vi "Read_Flatten.vi"(8 "error in":errorcluster, 11 "ChillerNew.lvclass":refnum<class "ChillerNew.lvclass">) -> (0 "error out":errorcluster, 2 "ReadValues":T1, 3 "output cluster":refnum<class "ChillerNew.lvclass">)   [LabVIEW 2023, in "ChillerNew.lvclass"]
uses:
  ChillerNew.lvclass
  ChillerNew.lvclass/ChillerNew.ctl
  9c8d422d-920d-4f62-ba29-e6a76558d5ae.vi
  9c8d422d-920d-4f62-ba29-e6a76558d5ae.vi/c28b0ead-42ad-4072-80a2-aca7f2bd7ce3.vi
  9c8d422d-920d-4f62-ba29-e6a76558d5ae.vi/219d0231-d98b-4193-b5cc-84f90e3c9091.vi
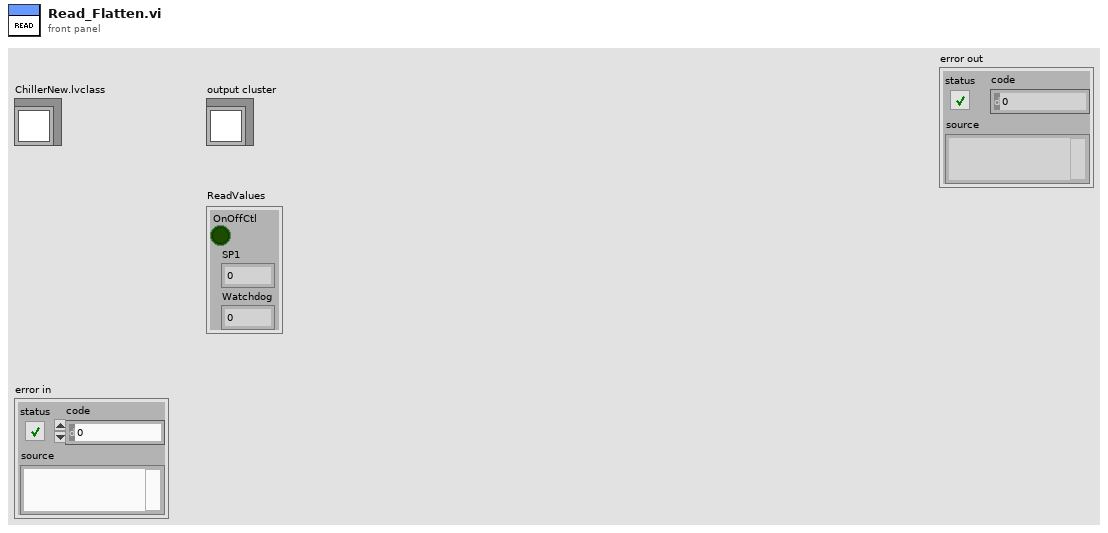
[diagram p1: front panel]
types:
  T1 = cluster{"OnOffCtl":bool, "SP1":dbl, "Watchdog":i32}
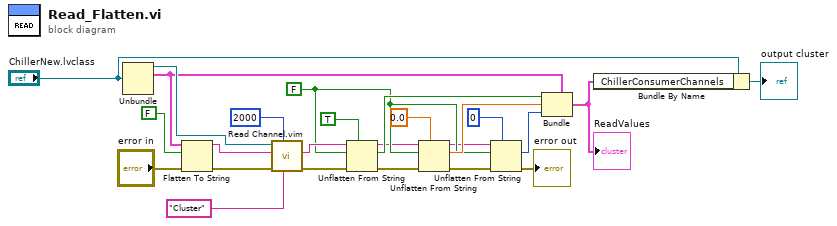
[diagram p0: block diagram]
diagram:
  w12 = FALSE ("data includes array or string size? (T)")
  n1 = Unbundle("ChillerNew.lvclass") -> (w25:refnum<k21>, w16:T1)  [unwired: 2 out]
  n2 = Flatten To String(anything=w16, prepend array or string size? (T)=FALSE, error in (no error)="error in") -> (data string=w19:string, error out=w3:errorcluster)  [unwired: 1 in, 1 out]
  n3 = call "Read Channel.vim"("Channel Type Description"="Cluster", "Timeout (ms)"=2000, "error in"=w3, "Data in"=w19, "ADAS HIL Channel in"=w25) -> ("error out"=w5:errorcluster, "Data out"=w18:string)  [unwired: 3 in, 2 out]
  n4 = Unflatten From String(type=TRUE, binary string=w18, data includes array or string size? (T)=w12, error in (no error)=w5) -> (rest of the binary string=w10:string, value=w15:bool, error out=w7:errorcluster)  [unwired: 1 in]
  n5 = Unflatten From String(type=0.0, binary string=w10, data includes array or string size? (T)=w12, error in (no error)=w7) -> (rest of the binary string=w11:string, value=w13:dbl, error out=w6:errorcluster)  [unwired: 1 in]
  n6 = Unflatten From String(type=0, binary string=w11, data includes array or string size? (T)=w12, error in (no error)=w6) -> (value=w8:i32, error out=→"error out":errorcluster)  [unwired: 1 in, 1 out]
  n7 = Bundle(cluster=w16, "OnOffCtl"=w15, "SP1"=w13, "Watchdog"=w8) -> (w1:T1)
  "ReadValues" <- w1
  n8 = Bundle By Name(cluster="ChillerNew.lvclass", "ChillerConsumerChannels"=w1) -> (→"output cluster":refnum<class "ChillerNew.lvclass">)
